vi "subtract_waveforms.vi"(8 "error in":errorcluster, 11 "Waveform array":waveform(dbl)[](array[waveform])) -> (0 "error out":errorcluster, 3 "Waveform out":waveform(dbl))   [LabVIEW 2020]
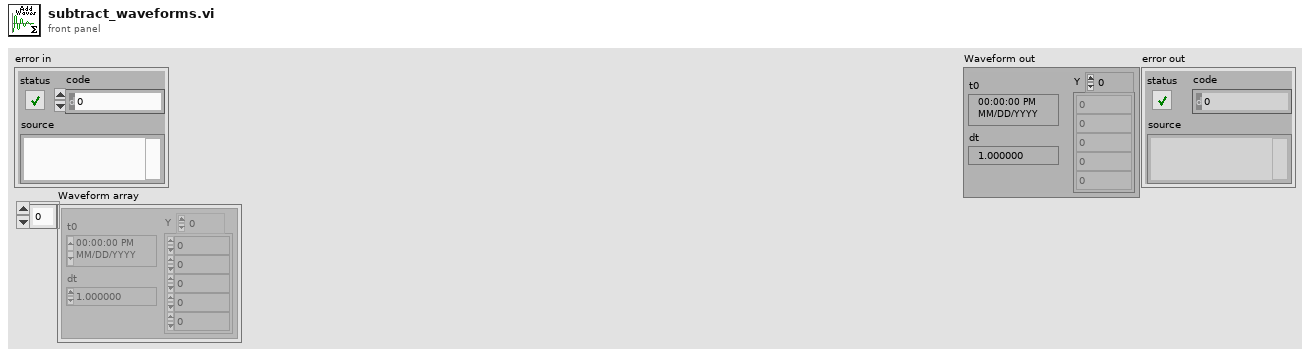
[diagram p1: front panel]
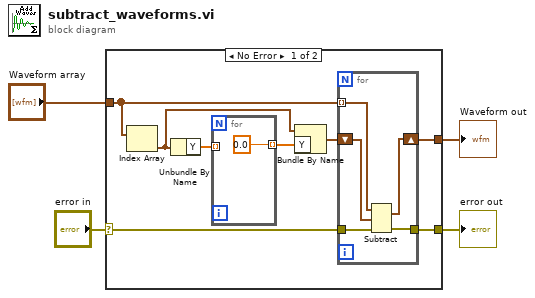
[diagram p0: block diagram]
diagram:
  n1 = case shown="No Error" "error in" {
    selector: "error in" -> [w8 w19]
    tunnel: "Waveform array" -> [w6 _]
    tunnel: [w7 w19] -> w1
    tunnel: [w5 _] -> w2
    frame No Error {
      n2 = Index Array(array=w6) -> (element=w10:waveform(dbl))  [unwired: 1 in]
      n3 = Unbundle By Name(w10) -> ("Y"=w12:dbl[])
      n4 = for {
        tunnel: w12 -> [_] mode=indexing
        tunnel: [0.0] -> w11 mode=indexing
      }
      n5 = Bundle By Name(cluster=w10, "Y"=w11) -> (w9:waveform(dbl))
      n6 = for {
        tunnel: w8 -> [w16]
        tunnel: [w15] -> w7
        tunnel: w6 -> [w14] mode=indexing
        shift-right: [w13] -> w5
        shift-left: w9 -> [w17]
        n7 = Subtract(1:w17, 2:w14, 4:w16) -> (0:w13:waveform(dbl), 3:w15:errorcluster)
      }
    }
    frame Error {
    }
  }
  "Waveform out" <- w2
  "error out" <- w1
